vi "Write RMS value.vi"(8 "error in (no error)":errorcluster, 10 "RMS value":dbl[unit] format="%0.2p", 11 "LHW-WfmBasicProperties in":refnum<class "LHW-WfmBasicProperties.lvclass">) -> (0 "error out":errorcluster, 3 "LHW-WfmBasicProperties out":refnum<class "LHW-WfmBasicProperties.lvclass">)   [LabVIEW 2016, in "LHW-Data.lvlib" / "LHW-WfmBasicProperties.lvclass"]
uses:
  LHW-WfmBasicProperties.lvclass
  LHW-WfmBasicProperties.lvclass/LHW-WfmBasicProperties.ctl
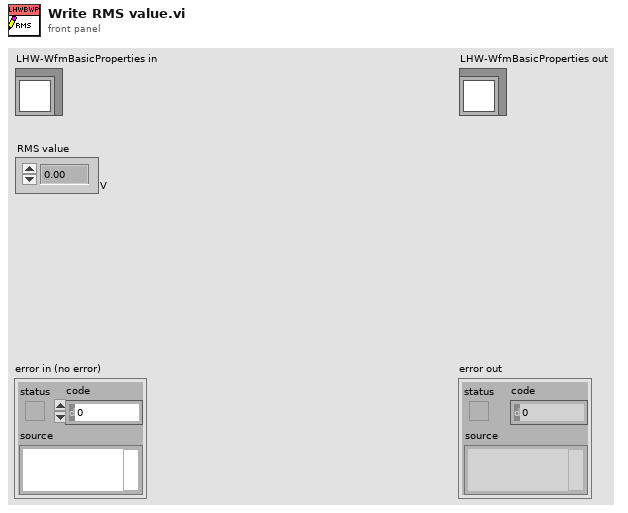
[diagram p1: front panel]
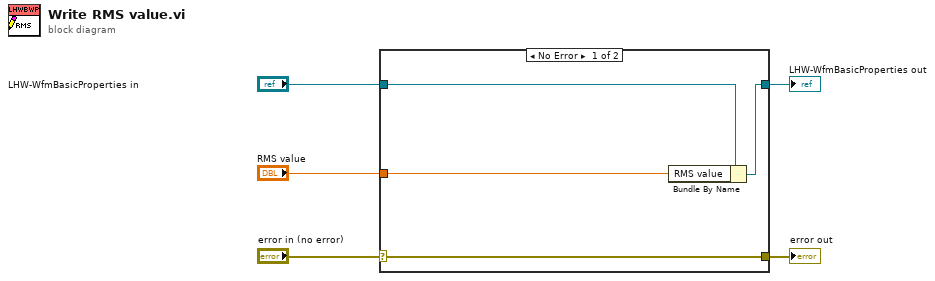
[diagram p0: block diagram]
diagram:
  n1 = case shown="No Error" "error in (no error)" {
    selector: "error in (no error)" -> [w9 w10]
    tunnel: [w9 w10] -> w4
    tunnel: [w7 w11] -> w2
    tunnel: "LHW-WfmBasicProperties in" -> [w8 w11]
    tunnel: "RMS value" -> [w6 _]
    frame No Error {
      n2 = Bundle By Name(cluster=w8, "RMS value"=w6) -> (w7:refnum<class "LHW-WfmBasicProperties.lvclass">)
    }
    frame Error {
    }
  }
  "error out" <- w4
  "LHW-WfmBasicProperties out" <- w2
